vi "UWV_DAQ_V1.0.vi"() -> ()   [LabVIEW 2018]
uses:
  <vilib>/DAQmx/read.llb/DAQmx Read (Analog 2D DBL NChan NSamp).vi
  <vilib>/DAQmx/create/channels.llb/DAQmx Create Channel (AI-Voltage-Basic).vi
  <vilib>/DAQmx/configure/timing.llb/DAQmx Timing (Sample Clock).vi
  <vilib>/DAQmx/miscellaneous.llb/DAQmx Fill In Error Info.vi
panel:
  in  "datalog path (use dialog)":path
  in  "save data":bool
  in  "stop":bool
  out "Waveform Graph":dbl[][](graph)
  in  "Record type":cluster{"Sampling rate":dbl, "Data":dbl[][]}
  in  "rate":dbl=1000.0 format="%0.2f"
  in  "physical channels":tag
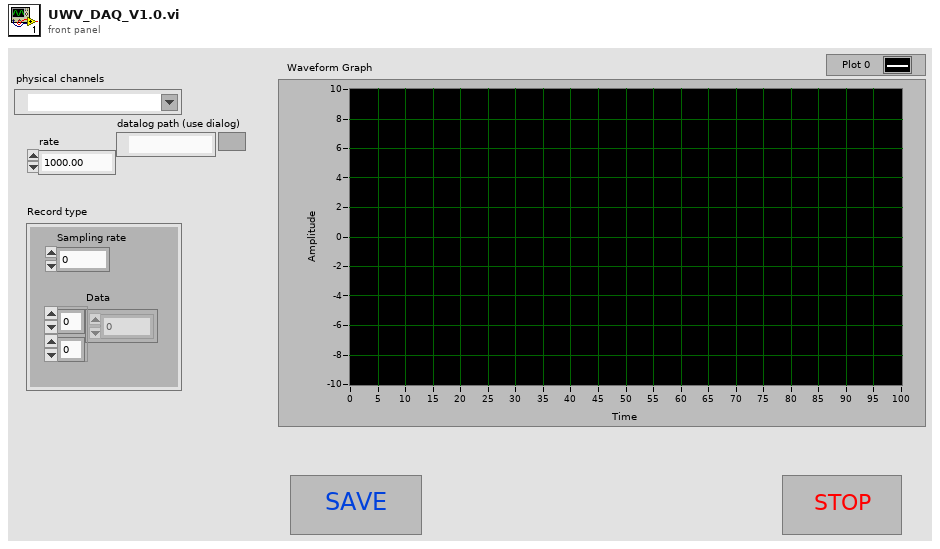
[diagram p1: front panel]
types:
  T1 = enum16{"open", "replace", "create", "open or create", "replace or create", "replace or create with confirmation"}
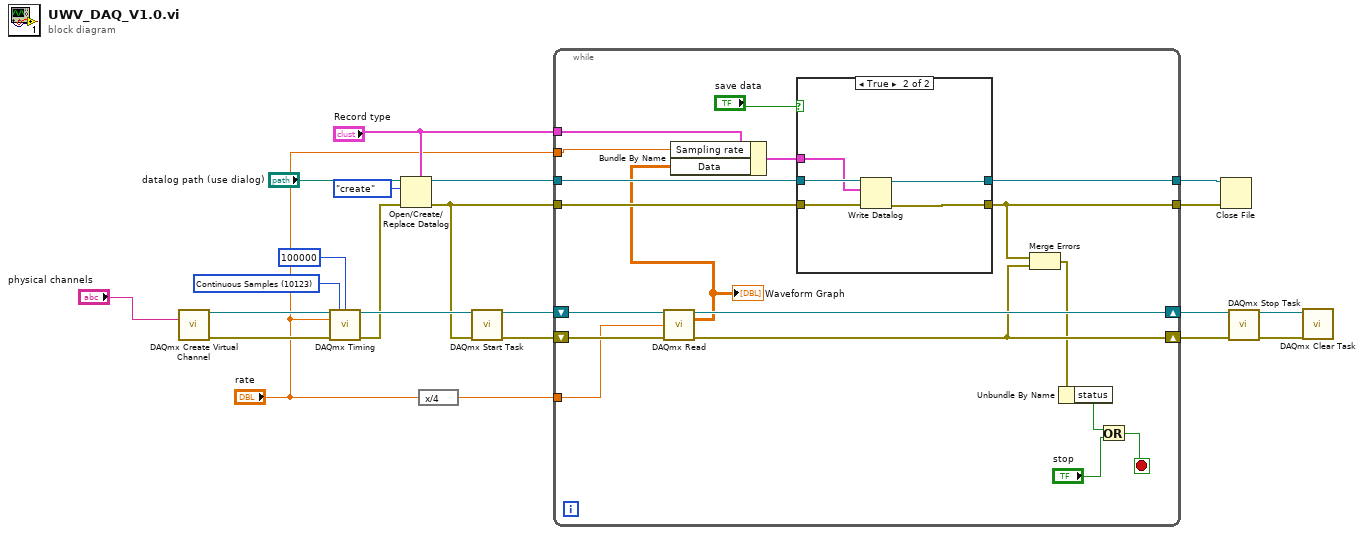
[diagram p0: block diagram]
diagram:
  w14 = 10123 items=["Finite Samples"=10178, "Continuous Samples"=10123, "Hardware Timed Single Point"=12522] ("sample mode")
  n1 = call-poly <vilib>:"DAQmx Create Virtual Channel.vi"("physical channels"="physical channels") -> ("task out"=w22:refnum<k21>, "error out"=w18:errorcluster)  [unwired: 13 in]
  n2 = call-poly <vilib>:"DAQmx Timing.vi"("task/channels in"=w22, "sample mode"=w14, "samples per channel"=100000, "rate"="rate", "error in"=w18) -> ("task out"=w21:refnum<k21>, "error out"=w9:errorcluster)  [unwired: 9 in]
  n3 = Open/Create/Replace Datalog(5:"Record type", 8:w9, 10:T1."create" ("operation (0:open)"), 11:"datalog path (use dialog)") -> (0:w8:errorcluster, 3:w10:refnum<k1>)  [unwired: 2 in, 1 out]
  n4 = expression code="x/4"("rate") -> (w7:dbl)
  n5 = call <vilib>:"DAQmx Start Task.vi"("task/channels in"=w21, "error in"=w8) -> ("task out"=w20:refnum<k21>, "error out"=w17:errorcluster)  [unwired: 12 in]
  n6 = while {
    shift-right: [w39] -> w19
    shift-left: w20 -> [w40]
    shift-right: [w28] -> w16
    shift-left: w17 -> [w38]
    tunnel: w10 -> [w36]
    tunnel: w8 -> [w35]
    tunnel: w7 -> [w37]
    tunnel: "Record type" -> [w34]
    tunnel: "rate" -> [w33]
    tunnel: [w29] -> w4
    tunnel: [w30] -> w3
    stop <- w26 stop-if-true
    n7 = call-poly <vilib>:"DAQmx Read.vi"("task/channels in"=w40, "number of samples per channel"=w37, "error in"=w38) -> ("task out"=w39:refnum<k21>, "data"=w32:dbl[][], "error out"=w28:errorcluster)  [unwired: 10 in]
    "Waveform Graph" <- w32
    n8 = Bundle By Name(cluster=w34, "Sampling rate"=w33, "Data"=w32) -> (w31:cluster{"Sampling rate":dbl, "Data":dbl[][]})
    n9 = case shown="True" "save data" {
      tunnel: w36 -> [w42 w46]
      tunnel: w35 -> [w41 w47]
      tunnel: [w42 w45] -> w30
      tunnel: [w41 w44] -> w29
      tunnel: w31 -> [_ w43]
      frame False {
      }
      frame True {
        n10 = Write Datalog(4:w47, 6:w43, 7:w46) -> (0:w44:errorcluster, 3:w45:refnum<k1>)
      }
    }
    n11 = Merge Errors(w29, w28) -> (w27:errorcluster)
    n12 = Unbundle By Name(w27) -> ("status"=w25:bool)
    n13 = Or(x=w25, y="stop") -> (x .or. y?=w26:bool)
  }
  n14 = Close File(refnum=w3, error in=w4) -> ()  [unwired: 2 out]
  n15 = call <vilib>:"DAQmx Stop Task.vi"("task/channels in"=w19, "error in"=w16) -> ("task out"=w12:refnum<k21>, "error out"=w11:errorcluster)  [unwired: 12 in]
  n16 = call <vilib>:"DAQmx Clear Task.vi"("task in"=w12, "error in"=w11) -> ()  [unwired: 13 in, 1 out]
